vi "FPGA_main_v2.vi"() -> ()   [LabVIEW 2020]
doc: "16 channels in NI9205, 16 channels in NI9208"
uses:
  <vilib>/LabVIEW Targets/FPGA/cRIO/shared/nicrio_ModuleControls/nicrio_cRIO-9205_TerminalMode.ctl
  <vilib>/LabVIEW Targets/FPGA/cRIO/shared/nicrio_ModuleControls/nicrio_cRIO-9205_VoltageRange.ctl
  <vilib>/LabVIEW Targets/FPGA/cRIO/shared/nicrio_ModuleControls/nicrio_BasicConversionTime.ctl
  <vilib>/rvi/Emulation/niFpgaGetClockAttributes.vi
  <vilib>/rvi/Emulation/niFpgaSctlEmulationGetInTimedLoop.vi
  <vilib>/rvi/Emulation/niFpgaEmulationReportErrorSimple.vi
  <vilib>/rvi/eio/common/nirviEmuTemplateMethod_errors.vi
  <vilib>/rvi/Emulation/niFpgaEmulationIsFPGAContextNoSignature.vi
  <vilib>/rvi/errors/niFpgaSetErrorForExecOnDevCompSimple.vi
  <vilib>/rvi/eio/common/nirviEmuReportErrorAndStop.vi
  <vilib>/rvi/DataTransferAndStorage/Container/Common/niFpgaContainerGetUniqueNameForEmu.vi
  <vilib>/rvi/FIFO/Fifo_Resource/nirvififoEmulationSetSize.vi
  <vilib>/rvi/FIFO/Fifo_Resource/nirviFifoEmulationQueueMgr.vi
  <instcachedir>/0/nirviFifoEmulationQueueMgr_E5CAEC123FF24DC58D834DCA3CDAA9B5.lvgen/nirviFifoEmulationQueueMgr_E5CAEC123FF24DC58D834DCA3CDAA9B5_007.vi
  <vilib>/rvi/FIFO/Fifo_Resource/nirvififoEmulationDetermineInputValidOut.vi
  <vilib>/rvi/FIFO/Fifo_Resource/nirvififoEmulationCreateLock.vi
  <vilib>/rvi/Emulation/niFpgaProcessEmulError.vi
  <vilib>/rvi/FIFO/Fifo_Resource/nirvififoEmulationObtainLock.vi
  <vilib>/rvi/FIFO/Fifo_Resource/nirvififoEmulationReleaseLock.vi
  <vilib>/rvi/occurrence/nirviWaitOnOccurrenceBase.vi
  <vilib>/rvi/errors/nirviReportUnexpectedCaseInternalError.vi
  <vilib>/rvi/errors/nirviReportUnexpectedCaseInternalError (U32).vi
  <vilib>/rvi/Emulation/niFpgaCriticalErrorInLSC.vi
  <vilib>/Utility/error.llb/Clear Errors.vi
  Components/MovingAverage/64ptMovingAvg.vi
  <instcachedir>/0/nirviFifoEmulationQueueMgr_E5CAEC123FF24DC58D834DCA3CDAA9B5.lvgen/nirviFifoEmulationQueueMgr_E5CAEC123FF24DC58D834DCA3CDAA9B5_010.vi
  <vilib>/rvi/eio/common/nirviEmuTemplatePropertySet_noerrors.vi
  <vilib>/rvi/DataTransferAndStorage/Container/Common/niFpgaContainerSetEmuInfo.vi
  <vilib>/eio/EIONode/EIONode.xnode
  <vilib>/rvi/DataTransferAndStorage/Container/XNode/niFpgaContainer.xnode
  <vilib>/rvi/FIFO/Fifo_Resource/nirvififoEmulationWrite.vi
  <vilib>/rvi/FIFO/Fifo_Resource/nirvififoEmulationRead.vi
  <vilib>/eio/EIOMethodNode/EIOMethodNode.xnode
  <vilib>/eio/EIOPropertyNode/EIOPropertyNode.xnode
  <vilib>/rvi/LocalResourceManager/LocalResourceManager.xnode
  <vilib>/rvi/eio/common/nirviEmuTemplatePropertyGet_errors.vi
  <vilib>/rvi/eio/common/nirviEmuTemplatePropertyGet_noerrors.vi
  <vilib>/rvi/eio/common/nirviEmuTemplatePropertySet_errors.vi
  Components/MovingAverage/MovingAvg.lvlib
panel:
  in  "NI9208 Sample Time [ms]":u32=31
  in  "NI9205 Sample Time [ticks]":u32=5120
  out "NI9208 AI proc. loop time [ms]":u32
  out "NI9208: AI15 [A]":fxp<+/-,24,-4> format="%#.6g"
  out "NI9208: AI14 [A]":fxp<+/-,24,-4> format="%#.6g"
  out "NI9208: AI13 [A]":fxp<+/-,24,-4> format="%#.6g"
  out "NI9208: AI12 [A]":fxp<+/-,24,-4> format="%#.6g"
  out "NI9208: AI11 [A]":fxp<+/-,24,-4> format="%#.6g"
  out "NI9208: AI10 [A]":fxp<+/-,24,-4> format="%#.6g"
  out "NI9208: AI9 [A]":fxp<+/-,24,-4> format="%#.6g"
  out "NI9208: AI8 [A]":fxp<+/-,24,-4> format="%#.6g"
  out "NI9208 FIFO\nOverflow?":bool
  out "NI9208 AI loop time [ms]":u32
  out "NI9208: AI7 [A]":fxp<+/-,24,-4> format="%#.6g"
  out "NI9208: AI6 [A]":fxp<+/-,24,-4> format="%#.6g"
  out "NI9208: AI5 [A]":fxp<+/-,24,-4> format="%#.6g"
  out "NI9208: AI4 [A]":fxp<+/-,24,-4> format="%#.6g"
  out "NI9208: AI3 [A]":fxp<+/-,24,-4> format="%#.6g"
  out "NI9208: AI2 [A]":fxp<+/-,24,-4> format="%#.6g"
  out "NI9208: AI1 [A]":fxp<+/-,24,-4> format="%#.6g"
  out "NI9208: AI0 [A]":fxp<+/-,24,-4> format="%#.6g"
  out "NI9205: AI23 [V]":fxp<+/-,35,5> format="%#.6g"
  out "NI9205: AI22 [V]":fxp<+/-,35,5> format="%#.6g"
  out "NI9205: AI21 [V]":fxp<+/-,35,5> format="%#.6g"
  out "NI9205: AI20 [V]":fxp<+/-,35,5> format="%#.6g"
  out "NI9205: AI19 [V]":fxp<+/-,35,5> format="%#.6g"
  out "NI9205: AI18 [V]":fxp<+/-,35,5> format="%#.6g"
  out "NI9205: AI17 [V]":fxp<+/-,35,5> format="%#.6g"
  out "NI9205: AI16 [V]":fxp<+/-,35,5> format="%#.6g"
  out "NI9205: AI7 [V]":fxp<+/-,35,5> format="%#.6g"
  out "NI9205: AI6 [V]":fxp<+/-,35,5> format="%#.6g"
  out "NI9205: AI5 [V]":fxp<+/-,35,5> format="%#.6g"
  out "NI9205: AI4 [V]":fxp<+/-,35,5> format="%#.6g"
  out "NI9205: AI3 [V]":fxp<+/-,35,5> format="%#.6g"
  out "NI9205: AI2 [V]":fxp<+/-,35,5> format="%#.6g"
  out "NI9205: AI1 [V]":fxp<+/-,35,5> format="%#.6g"
  out "NI9205: AI0 [V]":fxp<+/-,35,5> format="%#.6g"
  out "NI9205 AI proc. loop time [ticks]":u32
  out "NI9205 FIFO\nOverflow?":bool
  out "NI9205 AI loop time [ticks]":u32
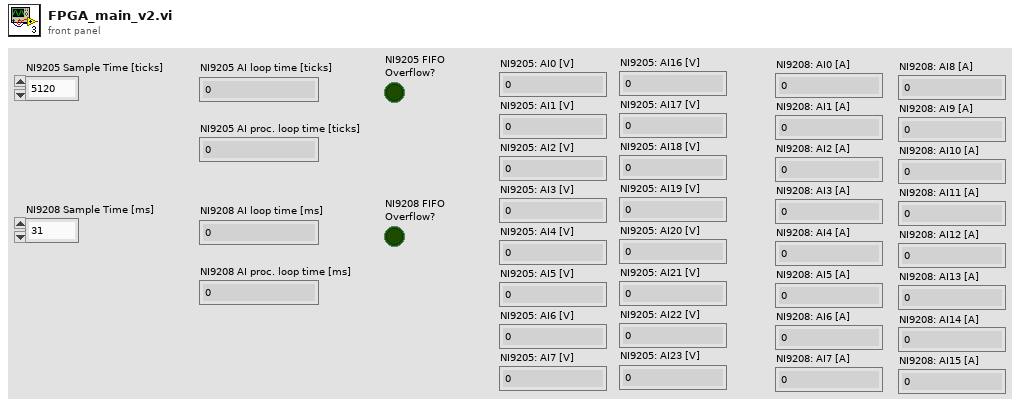
[diagram p1: front panel]
types:
  T1 = typedef "nicrio_BasicConversionTime.ctl" = enum8{"High Speed", "High Resolution"}
  T2 = typedef "nicrio_cRIO-9205_VoltageRange.ctl" = enum8{"+/- 10V", "+/- 5V", "+/- 1V", "+/- 200mV"}
  T3 = typedef "nicrio_cRIO-9205_TerminalMode.ctl" = enum8{"RSE", "NRSE", "DIFF"}
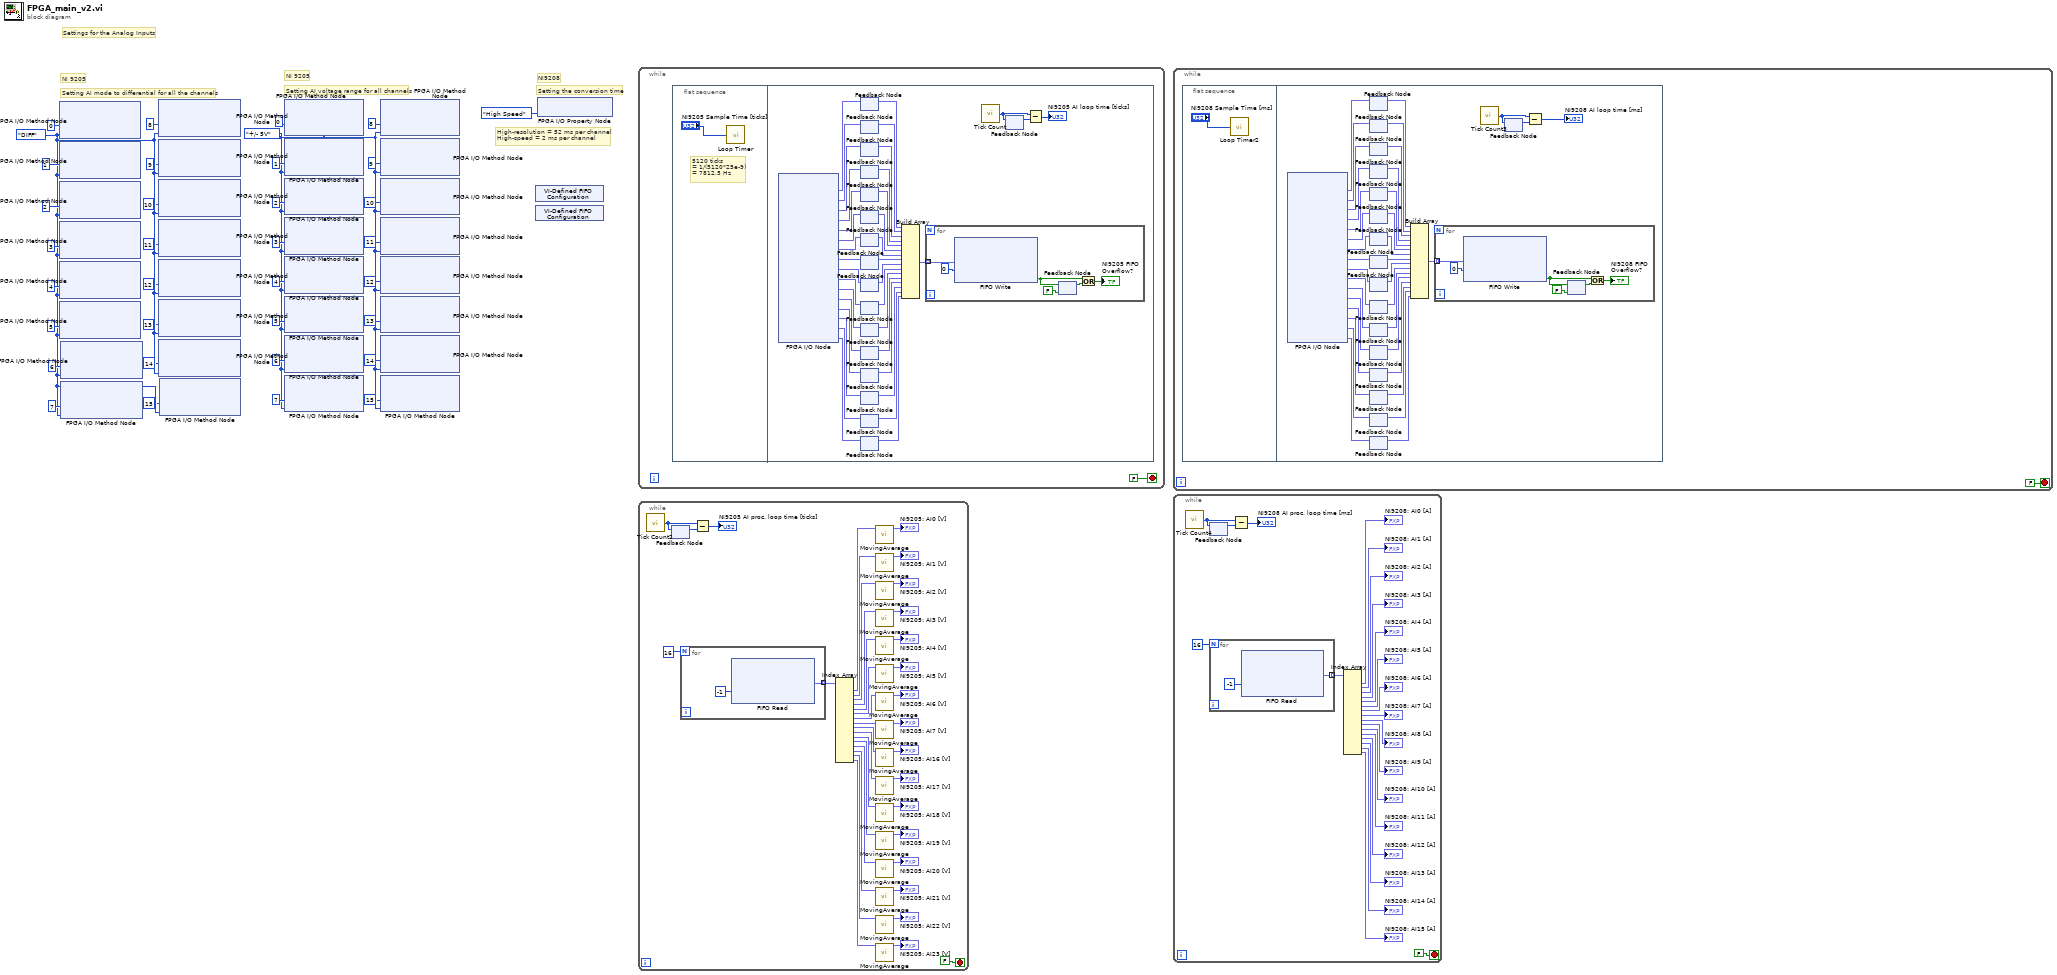
[diagram p0: block diagram]
diagram:
  w2 = nicrio_cRIO-9205_VoltageRange."+/- 5V" ("Voltage Range")
  w27 = nicrio_cRIO-9205_TerminalMode."DIFF" ("Terminal Mode")
  # "High-resolution = 52 ms per channel\nHigh-speed = 2 ms per channel"
  # "Setting the conversion time"
  # "NI9208"
  # "NI 9205"
  # "Setting AI voltage range for all channels"
  # "NI 9205"
  # "Setting AI mode to differential for all the channels"
  # "Settings for the Analog Inputs"
  n1 = xnode "FPGA I/O Method Node"("AI Channel"=u8 0, "Terminal Mode"=w27) -> ()  [unwired: 1 in, 1 out]
  n2 = xnode "FPGA I/O Method Node"("AI Channel"=u8 1, "Terminal Mode"=w27) -> ()  [unwired: 1 in, 1 out]
  n3 = xnode "FPGA I/O Method Node"("AI Channel"=u8 2, "Terminal Mode"=w27) -> ()  [unwired: 1 in, 1 out]
  n4 = xnode "FPGA I/O Method Node"("AI Channel"=u8 3, "Terminal Mode"=w27) -> ()  [unwired: 1 in, 1 out]
  n5 = xnode "FPGA I/O Method Node"("AI Channel"=u8 4, "Terminal Mode"=w27) -> ()  [unwired: 1 in, 1 out]
  n6 = xnode "FPGA I/O Method Node"("AI Channel"=u8 5, "Terminal Mode"=w27) -> ()  [unwired: 1 in, 1 out]
  n7 = xnode "FPGA I/O Method Node"("AI Channel"=u8 6, "Terminal Mode"=w27) -> ()  [unwired: 1 in, 1 out]
  n8 = xnode "FPGA I/O Method Node"("AI Channel"=u8 7, "Terminal Mode"=w27) -> ()  [unwired: 1 in, 1 out]
  n9 = xnode "FPGA I/O Method Node"("AI Channel"=u8 8, "Terminal Mode"=w27) -> ()  [unwired: 1 in, 1 out]
  n10 = xnode "FPGA I/O Method Node"("AI Channel"=u8 9, "Terminal Mode"=w27) -> ()  [unwired: 1 in, 1 out]
  n11 = xnode "FPGA I/O Method Node"("AI Channel"=u8 10, "Terminal Mode"=w27) -> ()  [unwired: 1 in, 1 out]
  n12 = xnode "FPGA I/O Method Node"("AI Channel"=u8 11, "Terminal Mode"=w27) -> ()  [unwired: 1 in, 1 out]
  n13 = xnode "FPGA I/O Method Node"("AI Channel"=u8 12, "Terminal Mode"=w27) -> ()  [unwired: 1 in, 1 out]
  n14 = xnode "FPGA I/O Method Node"("AI Channel"=u8 13, "Terminal Mode"=w27) -> ()  [unwired: 1 in, 1 out]
  n15 = xnode "FPGA I/O Method Node"("AI Channel"=u8 14, "Terminal Mode"=w27) -> ()  [unwired: 1 in, 1 out]
  n16 = xnode "FPGA I/O Method Node"("AI Channel"=u8 15, "Terminal Mode"=w27) -> ()  [unwired: 1 in, 1 out]
  n17 = xnode "FPGA I/O Method Node"("AI Channel"=u8 0, "Voltage Range"=w2) -> ()  [unwired: 1 in, 1 out]
  n18 = xnode "FPGA I/O Method Node"("AI Channel"=u8 1, "Voltage Range"=w2) -> ()  [unwired: 1 in, 1 out]
  n19 = xnode "FPGA I/O Method Node"("AI Channel"=u8 2, "Voltage Range"=w2) -> ()  [unwired: 1 in, 1 out]
  n20 = xnode "FPGA I/O Method Node"("AI Channel"=u8 3, "Voltage Range"=w2) -> ()  [unwired: 1 in, 1 out]
  n21 = xnode "FPGA I/O Method Node"("AI Channel"=u8 4, "Voltage Range"=w2) -> ()  [unwired: 1 in, 1 out]
  n22 = xnode "FPGA I/O Method Node"("AI Channel"=u8 5, "Voltage Range"=w2) -> ()  [unwired: 1 in, 1 out]
  n23 = xnode "FPGA I/O Method Node"("AI Channel"=u8 6, "Voltage Range"=w2) -> ()  [unwired: 1 in, 1 out]
  n24 = xnode "FPGA I/O Method Node"("AI Channel"=u8 7, "Voltage Range"=w2) -> ()  [unwired: 1 in, 1 out]
  n25 = xnode "FPGA I/O Method Node"("AI Channel"=u8 8, "Voltage Range"=w2) -> ()  [unwired: 1 in, 1 out]
  n26 = xnode "FPGA I/O Method Node"("AI Channel"=u8 9, "Voltage Range"=w2) -> ()  [unwired: 1 in, 1 out]
  n27 = xnode "FPGA I/O Method Node"("AI Channel"=u8 10, "Voltage Range"=w2) -> ()  [unwired: 1 in, 1 out]
  n28 = xnode "FPGA I/O Method Node"("AI Channel"=u8 11, "Voltage Range"=w2) -> ()  [unwired: 1 in, 1 out]
  n29 = xnode "FPGA I/O Method Node"("AI Channel"=u8 12, "Voltage Range"=w2) -> ()  [unwired: 1 in, 1 out]
  n30 = xnode "FPGA I/O Method Node"("AI Channel"=u8 13, "Voltage Range"=w2) -> ()  [unwired: 1 in, 1 out]
  n31 = xnode "FPGA I/O Method Node"("AI Channel"=u8 14, "Voltage Range"=w2) -> ()  [unwired: 1 in, 1 out]
  n32 = xnode "FPGA I/O Method Node"("AI Channel"=u8 15, "Voltage Range"=w2) -> ()  [unwired: 1 in, 1 out]
  n33 = xnode "VI-Defined FIFO Configuration"() -> ()  [unwired: 1 out]
  n34 = xnode "VI-Defined FIFO Configuration"() -> ()  [unwired: 1 out]
  n35 = xnode "FPGA I/O Property Node"("Conversion Time"=nicrio_BasicConversionTime."High Speed") -> ()  [unwired: 1 in, 1 out]
  n36 = while {
    stop <- FALSE stop-if-true
    n37 = flat-sequence {
      frame #0 {
        # "5120 ticks\n= 1/(5120*25e-9) \n= 7812.5 Hz"
        n38 = call "Loop Timer"("Count(Ticks)"="NI9205 Sample Time [ticks]") -> ()  [unwired: 1 out]
      }
      frame #1 {
        n39 = xnode "FPGA I/O Node"() -> ("Mod1/AI0"=w56:fxp<+/-,26,5>, "Mod1/AI1"=w55:fxp<+/-,26,5>, "Mod1/AI2"=w54:fxp<+/-,26,5>, "Mod1/AI3"=w53:fxp<+/-,26,5>, "Mod1/AI4"=w52:fxp<+/-,26,5>, "Mod1/AI5"=w51:fxp<+/-,26,5>, "Mod1/AI6"=w50:fxp<+/-,26,5>, "Mod1/AI7"=w49:fxp<+/-,26,5>, "Mod1/AI16"=w48:fxp<+/-,26,5>, "Mod1/AI17"=w47:fxp<+/-,26,5>, "Mod1/AI18"=w46:fxp<+/-,26,5>, "Mod1/AI19"=w45:fxp<+/-,26,5>, "Mod1/AI20"=w44:fxp<+/-,26,5>, "Mod1/AI21"=w43:fxp<+/-,26,5>, "Mod1/AI22"=w42:fxp<+/-,26,5>, "Mod1/AI23"=w41:fxp<+/-,26,5>)  [unwired: 16 in, 16 out]
        n40 = feedback #1() -> (w57:fxp<+/-,26,5>)  [unwired: 1 in]
        n41 = feedback-in #1(w56) -> ()
        n42 = feedback #2() -> (w58:fxp<+/-,26,5>)  [unwired: 1 in]
        n43 = feedback-in #2(w55) -> ()
        n44 = feedback #3() -> (w59:fxp<+/-,26,5>)  [unwired: 1 in]
        n45 = feedback-in #3(w54) -> ()
        n46 = feedback #4() -> (w60:fxp<+/-,26,5>)  [unwired: 1 in]
        n47 = feedback-in #4(w53) -> ()
        n48 = feedback #5() -> (w61:fxp<+/-,26,5>)  [unwired: 1 in]
        n49 = feedback-in #5(w52) -> ()
        n50 = feedback #6() -> (w62:fxp<+/-,26,5>)  [unwired: 1 in]
        n51 = feedback-in #6(w51) -> ()
        n52 = feedback #7() -> (w63:fxp<+/-,26,5>)  [unwired: 1 in]
        n53 = feedback-in #7(w50) -> ()
        n54 = feedback #8() -> (w64:fxp<+/-,26,5>)  [unwired: 1 in]
        n55 = feedback-in #8(w49) -> ()
        n56 = feedback #9() -> (w65:fxp<+/-,26,5>)  [unwired: 1 in]
        n57 = feedback-in #9(w48) -> ()
        n58 = feedback #10() -> (w66:fxp<+/-,26,5>)  [unwired: 1 in]
        n59 = feedback-in #10(w47) -> ()
        n60 = feedback #11() -> (w67:fxp<+/-,26,5>)  [unwired: 1 in]
        n61 = feedback-in #11(w46) -> ()
        n62 = feedback #12() -> (w68:fxp<+/-,26,5>)  [unwired: 1 in]
        n63 = feedback-in #12(w45) -> ()
        n64 = feedback #13() -> (w69:fxp<+/-,26,5>)  [unwired: 1 in]
        n65 = feedback-in #13(w44) -> ()
        n66 = feedback #14() -> (w70:fxp<+/-,26,5>)  [unwired: 1 in]
        n67 = feedback-in #14(w43) -> ()
        n68 = feedback #15() -> (w71:fxp<+/-,26,5>)  [unwired: 1 in]
        n69 = feedback-in #15(w42) -> ()
        n70 = feedback #16() -> (w72:fxp<+/-,26,5>)  [unwired: 1 in]
        n71 = feedback-in #16(w41) -> ()
        n72 = Build Array(w57, w58, w59, w60, w61, w62, w63, w64, w65, w66, w67, w68, w69, w70, w71, w72) -> (w73:fxp<+/-,26,5>[])
        n73 = for {
          tunnel: w73 -> [w79] mode=indexing
          n74 = xnode ("FIFO Write")("Element"=w79, "Timeout"=0) -> ("Timed Out?"=w74:bool)  [unwired: 1 in, 1 out]
          n75 = feedback #17(FALSE ("Timed Out?")) -> (w76:bool)
          n76 = feedback-in #17(w74) -> ()
          n77 = Or(x=w74, y=w76) -> (x .or. y?=→"NI9205 FIFO\nOverflow?":bool)
        }
        n78 = call "Tick Count"() -> ("Tick Count(Ticks)"=w38:u32)
        n79 = feedback #18() -> (w39:u32)  [unwired: 1 in]
        n80 = feedback-in #18(w38) -> ()
        n81 = Subtract(x=w38, y=w39) -> (x-y=→"NI9205 AI loop time [ticks]":u32)
      }
    }
  }
  n82 = while {
    stop <- FALSE stop-if-true
    n83 = call "Tick Count2"() -> ("Tick Count(Ticks)"=w116:u32)
    n84 = feedback #19() -> (w115:u32)  [unwired: 1 in]
    n85 = feedback-in #19(w116) -> ()
    n86 = for {
      N: 16 -> [_]
      tunnel: [w118] -> w113 mode=indexing
      n87 = xnode ("FIFO Read")("Timeout"=-1) -> ("Element"=w118:fxp<+/-,26,5>)  [unwired: 1 in, 2 out]
    }
    n88 = Subtract(x=w116, y=w115) -> (x-y=→"NI9205 AI proc. loop time [ticks]":u32)
    n89 = Index Array(array=w113) -> (element #1=w111:fxp<+/-,26,5>, element #2=w110:fxp<+/-,26,5>, element #3=w109:fxp<+/-,26,5>, element #4=w108:fxp<+/-,26,5>, element #5=w107:fxp<+/-,26,5>, element #6=w106:fxp<+/-,26,5>, element #7=w105:fxp<+/-,26,5>, element #8=w104:fxp<+/-,26,5>, element #9=w103:fxp<+/-,26,5>, element #10=w102:fxp<+/-,26,5>, element #11=w101:fxp<+/-,26,5>, element #12=w100:fxp<+/-,26,5>, element #13=w99:fxp<+/-,26,5>, element #14=w98:fxp<+/-,26,5>, element #15=w97:fxp<+/-,26,5>, element #16=w96:fxp<+/-,26,5>)  [unwired: 16 in]
    n90 = call-poly "MovingAverage.vi"("Raw input"=w111) -> ("Output"=→"NI9205: AI0 [V]":fxp<+/-,35,5>)  [unwired: 10 in]
    n91 = call-poly "MovingAverage.vi"("Raw input"=w110) -> ("Output"=→"NI9205: AI1 [V]":fxp<+/-,35,5>)  [unwired: 10 in]
    n92 = call-poly "MovingAverage.vi"("Raw input"=w109) -> ("Output"=→"NI9205: AI2 [V]":fxp<+/-,35,5>)  [unwired: 10 in]
    n93 = call-poly "MovingAverage.vi"("Raw input"=w108) -> ("Output"=→"NI9205: AI3 [V]":fxp<+/-,35,5>)  [unwired: 10 in]
    n94 = call-poly "MovingAverage.vi"("Raw input"=w107) -> ("Output"=→"NI9205: AI4 [V]":fxp<+/-,35,5>)  [unwired: 10 in]
    n95 = call-poly "MovingAverage.vi"("Raw input"=w106) -> ("Output"=→"NI9205: AI5 [V]":fxp<+/-,35,5>)  [unwired: 10 in]
    n96 = call-poly "MovingAverage.vi"("Raw input"=w105) -> ("Output"=→"NI9205: AI6 [V]":fxp<+/-,35,5>)  [unwired: 10 in]
    n97 = call-poly "MovingAverage.vi"("Raw input"=w104) -> ("Output"=→"NI9205: AI7 [V]":fxp<+/-,35,5>)  [unwired: 10 in]
    n98 = call-poly "MovingAverage.vi"("Raw input"=w103) -> ("Output"=→"NI9205: AI16 [V]":fxp<+/-,35,5>)  [unwired: 10 in]
    n99 = call-poly "MovingAverage.vi"("Raw input"=w102) -> ("Output"=→"NI9205: AI17 [V]":fxp<+/-,35,5>)  [unwired: 10 in]
    n100 = call-poly "MovingAverage.vi"("Raw input"=w101) -> ("Output"=→"NI9205: AI18 [V]":fxp<+/-,35,5>)  [unwired: 10 in]
    n101 = call-poly "MovingAverage.vi"("Raw input"=w100) -> ("Output"=→"NI9205: AI19 [V]":fxp<+/-,35,5>)  [unwired: 10 in]
    n102 = call-poly "MovingAverage.vi"("Raw input"=w99) -> ("Output"=→"NI9205: AI20 [V]":fxp<+/-,35,5>)  [unwired: 10 in]
    n103 = call-poly "MovingAverage.vi"("Raw input"=w98) -> ("Output"=→"NI9205: AI21 [V]":fxp<+/-,35,5>)  [unwired: 10 in]
    n104 = call-poly "MovingAverage.vi"("Raw input"=w97) -> ("Output"=→"NI9205: AI22 [V]":fxp<+/-,35,5>)  [unwired: 10 in]
    n105 = call-poly "MovingAverage.vi"("Raw input"=w96) -> ("Output"=→"NI9205: AI23 [V]":fxp<+/-,35,5>)  [unwired: 10 in]
  }
  n106 = while {
    stop <- FALSE stop-if-true
    n107 = flat-sequence {
      frame #0 {
        n108 = call "Loop Timer2"("Count(mSec)"="NI9208 Sample Time [ms]") -> ()  [unwired: 1 out]
      }
      frame #1 {
        n109 = xnode "FPGA I/O Node"() -> ("Mod2/AI0"=w140:fxp<+/-,24,-4>, "Mod2/AI1"=w139:fxp<+/-,24,-4>, "Mod2/AI2"=w138:fxp<+/-,24,-4>, "Mod2/AI3"=w137:fxp<+/-,24,-4>, "Mod2/AI4"=w136:fxp<+/-,24,-4>, "Mod2/AI5"=w135:fxp<+/-,24,-4>, "Mod2/AI6"=w134:fxp<+/-,24,-4>, "Mod2/AI7"=w133:fxp<+/-,24,-4>, "Mod2/AI8"=w132:fxp<+/-,24,-4>, "Mod2/AI9"=w131:fxp<+/-,24,-4>, "Mod2/AI10"=w130:fxp<+/-,24,-4>, "Mod2/AI11"=w129:fxp<+/-,24,-4>, "Mod2/AI12"=w128:fxp<+/-,24,-4>, "Mod2/AI13"=w127:fxp<+/-,24,-4>, "Mod2/AI14"=w126:fxp<+/-,24,-4>, "Mod2/AI15"=w125:fxp<+/-,24,-4>)  [unwired: 16 in, 16 out]
        n110 = feedback #20() -> (w142:fxp<+/-,24,-4>)  [unwired: 1 in]
        n111 = feedback-in #20(w140) -> ()
        n112 = feedback #21() -> (w143:fxp<+/-,24,-4>)  [unwired: 1 in]
        n113 = feedback-in #21(w139) -> ()
        n114 = feedback #22() -> (w144:fxp<+/-,24,-4>)  [unwired: 1 in]
        n115 = feedback-in #22(w138) -> ()
        n116 = feedback #23() -> (w145:fxp<+/-,24,-4>)  [unwired: 1 in]
        n117 = feedback-in #23(w137) -> ()
        n118 = feedback #24() -> (w146:fxp<+/-,24,-4>)  [unwired: 1 in]
        n119 = feedback-in #24(w136) -> ()
        n120 = feedback #25() -> (w147:fxp<+/-,24,-4>)  [unwired: 1 in]
        n121 = feedback-in #25(w135) -> ()
        n122 = feedback #26() -> (w148:fxp<+/-,24,-4>)  [unwired: 1 in]
        n123 = feedback-in #26(w134) -> ()
        n124 = feedback #27() -> (w149:fxp<+/-,24,-4>)  [unwired: 1 in]
        n125 = feedback-in #27(w133) -> ()
        n126 = feedback #28() -> (w150:fxp<+/-,24,-4>)  [unwired: 1 in]
        n127 = feedback-in #28(w132) -> ()
        n128 = feedback #29() -> (w151:fxp<+/-,24,-4>)  [unwired: 1 in]
        n129 = feedback-in #29(w131) -> ()
        n130 = feedback #30() -> (w152:fxp<+/-,24,-4>)  [unwired: 1 in]
        n131 = feedback-in #30(w130) -> ()
        n132 = feedback #31() -> (w153:fxp<+/-,24,-4>)  [unwired: 1 in]
        n133 = feedback-in #31(w129) -> ()
        n134 = feedback #32() -> (w154:fxp<+/-,24,-4>)  [unwired: 1 in]
        n135 = feedback-in #32(w128) -> ()
        n136 = feedback #33() -> (w155:fxp<+/-,24,-4>)  [unwired: 1 in]
        n137 = feedback-in #33(w127) -> ()
        n138 = feedback #34() -> (w156:fxp<+/-,24,-4>)  [unwired: 1 in]
        n139 = feedback-in #34(w126) -> ()
        n140 = feedback #35() -> (w157:fxp<+/-,24,-4>)  [unwired: 1 in]
        n141 = feedback-in #35(w125) -> ()
        n142 = Build Array(w142, w143, w144, w145, w146, w147, w148, w149, w150, w151, w152, w153, w154, w155, w156, w157) -> (w141:fxp<+/-,24,-4>[])
        n143 = for {
          tunnel: w141 -> [w163] mode=indexing
          n144 = xnode ("FIFO Write")("Element"=w163, "Timeout"=0) -> ("Timed Out?"=w158:bool)  [unwired: 1 in, 1 out]
          n145 = feedback #36(FALSE ("Timed Out?")) -> (w160:bool)
          n146 = feedback-in #36(w158) -> ()
          n147 = Or(x=w158, y=w160) -> (x .or. y?=→"NI9208 FIFO\nOverflow?":bool)
        }
        n148 = call "Tick Count3"() -> ("Tick Count(mSec)"=w122:u32)
        n149 = feedback #37() -> (w123:u32)  [unwired: 1 in]
        n150 = feedback-in #37(w122) -> ()
        n151 = Subtract(x=w122, y=w123) -> (x-y=→"NI9208 AI loop time [ms]":u32)
      }
    }
  }
  n152 = while {
    stop <- FALSE stop-if-true
    n153 = call "Tick Count4"() -> ("Tick Count(mSec)"=w166:u32)
    n154 = for {
      N: 16 -> [_]
      tunnel: [w186] -> w183 mode=indexing
      n155 = xnode ("FIFO Read")("Timeout"=-1) -> ("Element"=w186:fxp<+/-,24,-4>)  [unwired: 1 in, 2 out]
    }
    n156 = feedback #38() -> (w165:u32)  [unwired: 1 in]
    n157 = feedback-in #38(w166) -> ()
    n158 = Subtract(x=w166, y=w165) -> (x-y=→"NI9208 AI proc. loop time [ms]":u32)
    n159 = Index Array(array=w183) -> (element #1=→"NI9208: AI0 [A]":fxp<+/-,24,-4>, element #2=→"NI9208: AI1 [A]":fxp<+/-,24,-4>, element #3=→"NI9208: AI2 [A]":fxp<+/-,24,-4>, element #4=→"NI9208: AI3 [A]":fxp<+/-,24,-4>, element #5=→"NI9208: AI4 [A]":fxp<+/-,24,-4>, element #6=→"NI9208: AI5 [A]":fxp<+/-,24,-4>, element #7=→"NI9208: AI6 [A]":fxp<+/-,24,-4>, element #8=→"NI9208: AI7 [A]":fxp<+/-,24,-4>, element #9=→"NI9208: AI8 [A]":fxp<+/-,24,-4>, element #10=→"NI9208: AI9 [A]":fxp<+/-,24,-4>, element #11=→"NI9208: AI10 [A]":fxp<+/-,24,-4>, element #12=→"NI9208: AI11 [A]":fxp<+/-,24,-4>, element #13=→"NI9208: AI12 [A]":fxp<+/-,24,-4>, element #14=→"NI9208: AI13 [A]":fxp<+/-,24,-4>, element #15=→"NI9208: AI14 [A]":fxp<+/-,24,-4>, element #16=→"NI9208: AI15 [A]":fxp<+/-,24,-4>)  [unwired: 16 in]
  }
